vi "aggregate weekly.vi"(11 "Array":u32[](array[numeric])) -> (2 "array index":i32[](array[numeric]), 3 "weekly":u32[](array[numeric]))   [LabVIEW 2019]
panel:
  out "XY Graph":cluster{i32[], u32[]}(graph)
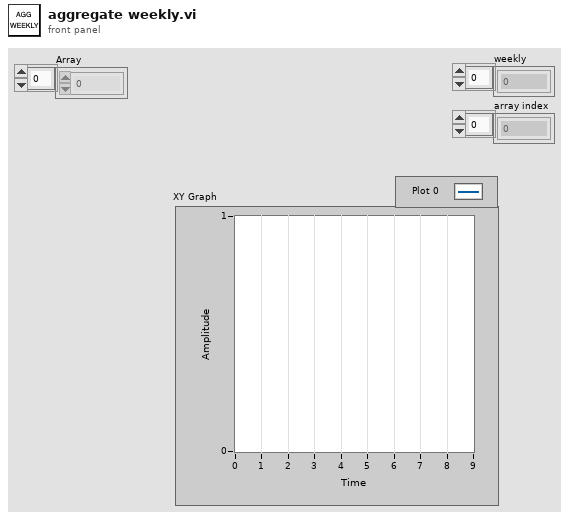
[diagram p1: front panel]
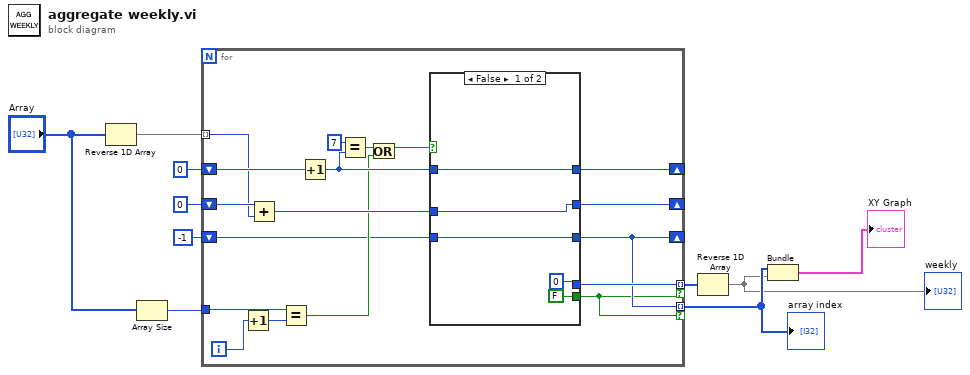
[diagram p0: block diagram]
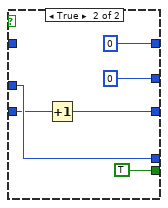
[diagram p2: hidden frame]
diagram:
  n1 = Reverse 1D Array(array="Array") -> (reversed array=w7:u32[])
  n2 = Array Size(array="Array") -> (size(s)=w3:i32)
  n3 = for {
    tunnel: w7 -> [w26] mode=indexing
    tunnel: [w19] -> w10 mode=indexing if=w11
    tunnel: [w12] -> w9 mode=indexing if=w11
    shift-right: [w23] -> _
    shift-left: 0 -> [w28]
    shift-right: [w22] -> _
    shift-left: 0 -> [w27]
    tunnel: w3 -> [w17]
    shift-right: [w12] -> _
    shift-left: -1 -> [w13]
    i -> [w16]
    n4 = Increment(x=w16) -> (x+1=w15:i32)
    n5 = Add(x=w27, y=w26) -> (x+y=w20:u32)
    n6 = Equal?(x=w17, y=w15) -> (x = y?=w14:bool)
    n7 = Increment(x=w28) -> (x+1=w21:i32)
    n8 = Equal?(x=7, y=w21) -> (x = y?=w24:bool)
    n9 = Or(x=w24, y=w14) -> (x .or. y?=w18:bool)
    n10 = case shown="False" w18 {
      tunnel: [w33 0] -> w23
      tunnel: [w32 0] -> w22
      tunnel: w21 -> [w33 _]
      tunnel: w20 -> [w32 w37]
      tunnel: [u32 0 w37] -> w19
      tunnel: [FALSE TRUE] -> w11
      tunnel: w13 -> [w29 w35]
      tunnel: [w29 w34] -> w12
      frame False {
      }
      frame True {
        n11 = Increment(x=w35) -> (x+1=w34:i32)
      }
    }
  }
  "array index" <- w9
  n12 = Reverse 1D Array(array=w10) -> (reversed array=w1:u32[])
  "weekly" <- w1
  n13 = Bundle(w9, w1) -> (→"XY Graph":cluster{i32[], u32[]})  [unwired: 1 in]
